vi "Slack-Read Config.vi"(0 "AppName":path, 11 "Error In":errorcluster) -> (4 "config":T2, 8 "users":T1[](array[typedef]), 15 "error out":errorcluster)   [LabVIEW 2020]
uses:
  Typedefs/Slack-Configuration.ctl
  Typedefs/Slack-User.ctl
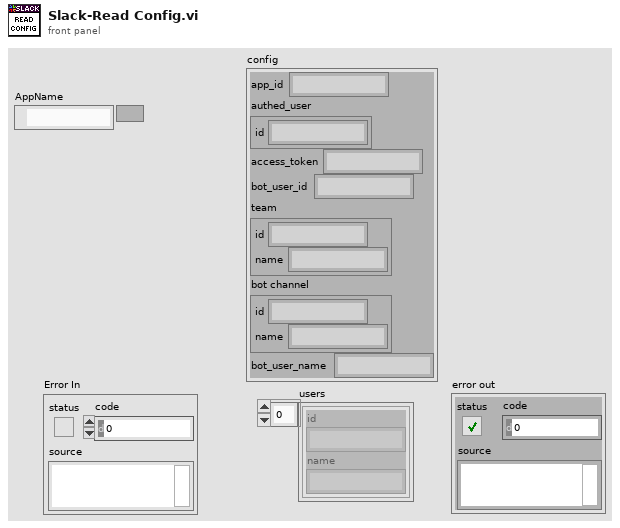
[diagram p1: front panel]
types:
  T1 = typedef "Slack-User.ctl" = cluster{"id":string, "name":string}
  T2 = typedef "Slack-Configuration.ctl" = cluster{"app_id":string, "authed_user":cluster{"id":string}, "access_token":string, "bot_user_id":string, "team":cluster{"id":string, "name":string}, "bot channel":cluster{"id":string, "name":string}, "bot_user_name":string}
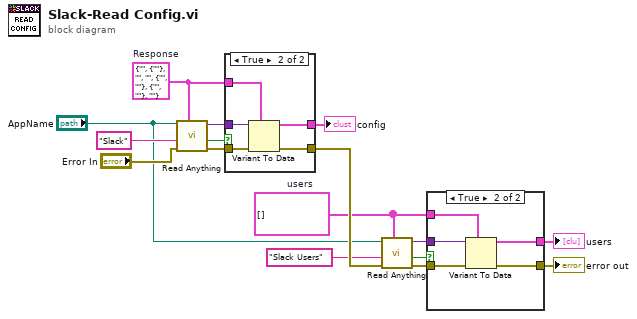
[diagram p0: block diagram]
diagram:
  w3 = T1[] []  # users
  w13 = T2 {"app_id"="", "authed_user"={"id"=""}, "access_token"="", "bot_user_id"="", "team"={"id"="", "name"=""}, "bot channel"={"id"="", "name"=""}, "bot_user_name"=""}  # Response
  n1 = call "Read Anything.vi"("Type of Anything"=w13, "Error In"="Error In", "Section Name (Name of \"Type of Anything\")"="Slack" ("Section Name (Name of \"Type of Anything\")"), "Path (dialog)"="AppName") -> ("Error Out"=w15:errorcluster, "Found?"=w11:bool, "Anything"=w14:variant)  [unwired: 5 in]
  n2 = case shown="True" w11 {
    tunnel: w15 -> [w17 w23]
    tunnel: w14 -> [_ w22]
    tunnel: w13 -> [w18 w21]
    tunnel: [w18 w20] -> w12
    tunnel: [w17 w19] -> w9
    frame False {
    }
    frame True {
      n3 = Variant To Data(error in=w23, type=w21, Variant=w22) -> (data=w20:T2, error out=w19:errorcluster)
    }
  }
  "config" <- w12
  n4 = call "Read Anything.vi"("Type of Anything"=w3, "Error In"=w9, "Section Name (Name of \"Type of Anything\")"="Slack Users" ("Section Name (Name of \"Type of Anything\")"), "Path (dialog)"="AppName") -> ("Error Out"=w6:errorcluster, "Found?"=w5:bool, "Anything"=w4:variant)  [unwired: 5 in]
  n5 = case shown="True" w5 {
    tunnel: w6 -> [w25 w30]
    tunnel: w4 -> [_ w29]
    tunnel: w3 -> [w24 w28]
    tunnel: [w25 w27] -> w2
    tunnel: [w24 w26] -> w1
    frame False {
    }
    frame True {
      n6 = Variant To Data(error in=w30, type=w28, Variant=w29) -> (data=w26:T1[], error out=w27:errorcluster)
    }
  }
  "error out" <- w2
  "users" <- w1
